vi "Find caller VI thats in project.vi"(8 "error in":errorcluster, 10 "All VIs in .proj":string[](array[string]), 11 "VI Refnum":refnum<vi>) -> (0 "error out":errorcluster, 1 "Parent Project VI":string, 2 "Parent found?":bool, 3 "VI Refnum (dup)":refnum<vi>, 4 "Parent Project VI Path":path, 5 "VI details":T1)   [LabVIEW 2013]
doc: "This .vi will search the project vis for a caller that's in the project. This is useful to find what vi is calling a dependency."
uses:
  Dependency cluster.ctl
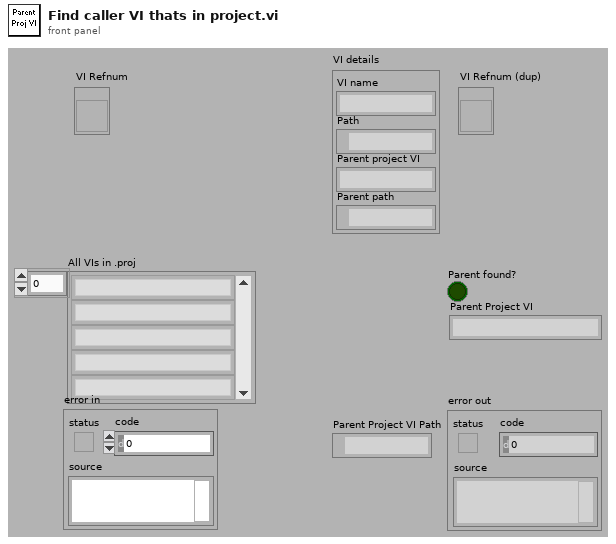
[diagram p1: front panel]
types:
  T1 = typedef "Dependency cluster.ctl" = cluster{"VI name":string, "Path":path, "Parent project VI":string, "Parent path":path}
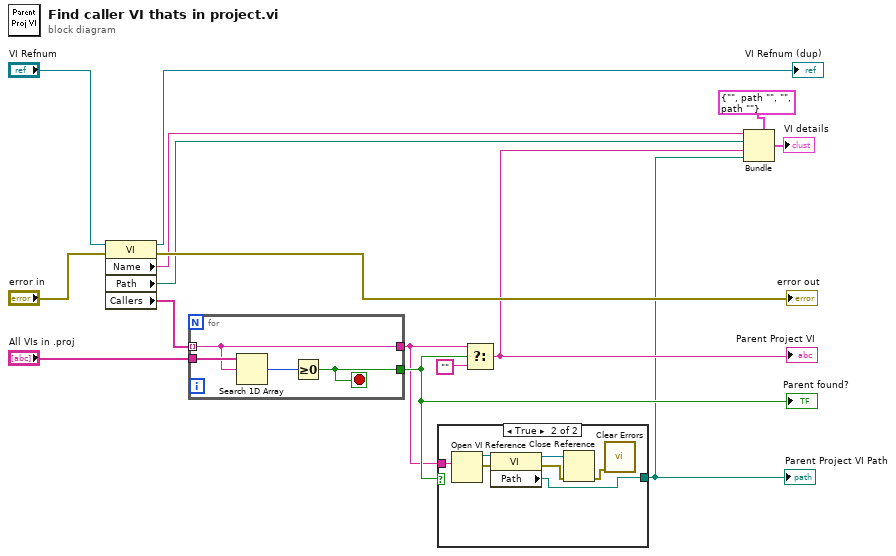
[diagram p0: block diagram]
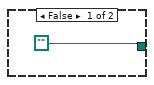
[diagram p2: hidden frame]
diagram:
  n1 = property class="VI"(reference="VI Refnum", error in="error in") -> (reference out=→"VI Refnum (dup)":refnum<vi>, error out=→"error out":errorcluster, "Name"=w5:string, "Path"=w4:path, "Callers"=w15:string[])
  n2 = for {
    tunnel: w15 -> [w16] mode=indexing
    tunnel: "All VIs in .proj" -> [w19]
    tunnel: [w18] -> w8
    tunnel: [w16] -> w7
    stop <- w18 stop-if-true
    n3 = Search 1D Array(1D array=w19, element=w16) -> (index of element=w17:i32)  [unwired: 1 out]
    n4 = Greater Or Equal To 0?(x=w17) -> (x >= 0?=w18:bool)
  }
  "Parent found?" <- w8
  n5 = case shown="True" w8 {
    tunnel: [path "" w25] -> w2
    tunnel: w7 -> [_ w22]
    frame False {
    }
    frame True {
      n6 = Open VI Reference(vi path=w22) -> (vi reference=w27:refnum<vi>, error out=w26:errorcluster)  [unwired: 1 in, 4 out]
      n7 = property class="VI"(reference=w27, error in=w26) -> (reference out=w23:refnum<vi>, error out=w24:errorcluster, "Path"=w25:path)
      n8 = Close Reference(reference=w23, error in (no error)=w24) -> (error out=w21:errorcluster)
      n9 = call <vilib>:"Clear Errors.vi"("error in (no error)"=w21) -> ()  [unwired: 7 out]
    }
  }
  "Parent Project VI Path" <- w2
  n10 = Select(t=w7, s=w8, f="") -> (s? t:f=w3:string)
  "Parent Project VI" <- w3
  n11 = Bundle(cluster=T1 {"VI name"="", "Path"=path "", "Parent project VI"="", "Parent path"=path ""}, "VI name"=w5, "Path"=w4, "Parent project VI"=w3, "Parent path"=w2) -> (→"VI details":T1)
